vi "Dallas simple relay switch.vi"() -> ()   [LabVIEW 2009]
uses:
  <vilib>/DAQmx/write.llb/DAQmx Write (Digital Bool 1Line 1Point).vi
  <vilib>/DAQmx/create/channels.llb/DAQmx Create Channel (DO-Digital Output).vi
panel:
  in  "stop":bool
  in  "wait (ms)":dbl
  in  "On (ms)":dbl
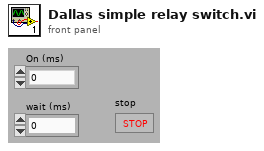
[diagram p1: front panel]
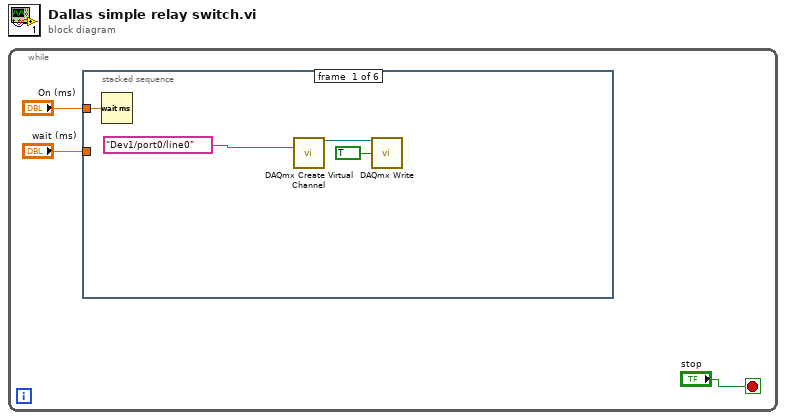
[diagram p0: block diagram]
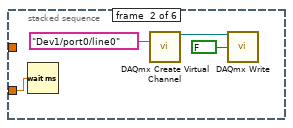
[diagram p2: hidden frame]
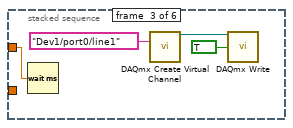
[diagram p3: hidden frame]
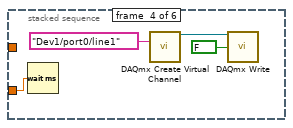
[diagram p4: hidden frame]
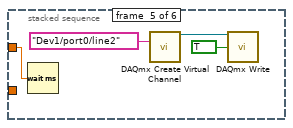
[diagram p5: hidden frame]
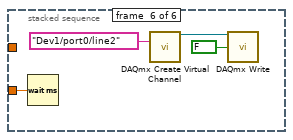
[diagram p6: hidden frame]
diagram:
  n1 = while {
    stop <- "stop" stop-if-true
    n2 = stacked-sequence {
      tunnel: "On (ms)" -> [w4 _ w12 _ w20 _]
      tunnel: "wait (ms)" -> [_ w8 _ w16 _ w24]
      frame #0 {
        n3 = Wait (ms)(milliseconds to wait=w4) -> ()  [unwired: 1 out]
        n4 = call-poly <vilib>:"DAQmx Create Virtual Channel.vi"("lines"=tag "Dev1/port0/line0") -> ("task out"=w6:refnum<k21>)  [unwired: 5 in, 9 out]
        n5 = call-poly <vilib>:"DAQmx Write.vi"("task/channels in"=w6, "data"=TRUE) -> ()  [unwired: 2 in, 12 out]
      }
      frame #1 {
        n6 = Wait (ms)(milliseconds to wait=w8) -> ()  [unwired: 1 out]
        n7 = call-poly <vilib>:"DAQmx Create Virtual Channel.vi"("lines"=tag "Dev1/port0/line0") -> ("task out"=w10:refnum<k21>)  [unwired: 5 in, 9 out]
        n8 = call-poly <vilib>:"DAQmx Write.vi"("task/channels in"=w10, "data"=FALSE) -> ()  [unwired: 2 in, 12 out]
      }
      frame #2 {
        n9 = Wait (ms)(milliseconds to wait=w12) -> ()  [unwired: 1 out]
        n10 = call-poly <vilib>:"DAQmx Create Virtual Channel.vi"("lines"=tag "Dev1/port0/line1") -> ("task out"=w14:refnum<k21>)  [unwired: 5 in, 9 out]
        n11 = call-poly <vilib>:"DAQmx Write.vi"("task/channels in"=w14, "data"=TRUE) -> ()  [unwired: 2 in, 12 out]
      }
      frame #3 {
        n12 = Wait (ms)(milliseconds to wait=w16) -> ()  [unwired: 1 out]
        n13 = call-poly <vilib>:"DAQmx Create Virtual Channel.vi"("lines"=tag "Dev1/port0/line1") -> ("task out"=w18:refnum<k21>)  [unwired: 5 in, 9 out]
        n14 = call-poly <vilib>:"DAQmx Write.vi"("task/channels in"=w18, "data"=FALSE) -> ()  [unwired: 2 in, 12 out]
      }
      frame #4 {
        n15 = Wait (ms)(milliseconds to wait=w20) -> ()  [unwired: 1 out]
        n16 = call-poly <vilib>:"DAQmx Create Virtual Channel.vi"("lines"=tag "Dev1/port0/line2") -> ("task out"=w22:refnum<k21>)  [unwired: 5 in, 9 out]
        n17 = call-poly <vilib>:"DAQmx Write.vi"("task/channels in"=w22, "data"=TRUE) -> ()  [unwired: 2 in, 12 out]
      }
      frame #5 {
        n18 = Wait (ms)(milliseconds to wait=w24) -> ()  [unwired: 1 out]
        n19 = call-poly <vilib>:"DAQmx Create Virtual Channel.vi"("lines"=tag "Dev1/port0/line2") -> ("task out"=w26:refnum<k21>)  [unwired: 5 in, 9 out]
        n20 = call-poly <vilib>:"DAQmx Write.vi"("task/channels in"=w26, "data"=FALSE) -> ()  [unwired: 2 in, 12 out]
      }
    }
  }
